vi "modbusTimestampInstruction.vi"(8 "error in (no error)":errorcluster, 11 "Model in":refnum<class "Model.lvclass">) -> (0 "error out":errorcluster, 3 "Model out":refnum<class "Model.lvclass">)   [LabVIEW 2016, in "Model.lvclass"]
uses:
  Model.lvclass
  Model.lvclass/Model.ctl
  ILCCommunications/ILCCommunications.lvclass
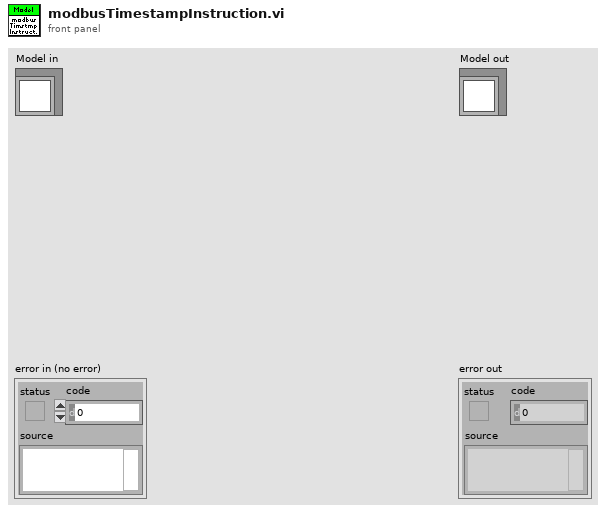
[diagram p1: front panel]
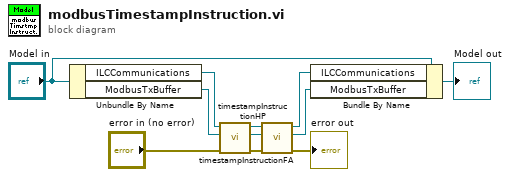
[diagram p0: block diagram]
diagram:
  n1 = Unbundle By Name("Model in") -> ("ILCCommunications"=w9:refnum<class "ILCCommunications.lvclass">, "ModbusTxBuffer"=w8:refnum<class "ModbusBuffer.lvclass">)
  n2 = call "timestampInstructionHP.vi"("error in (no error)"="error in (no error)", "ModbusBuffer in"=w8, "ILCCommunications in"=w9) -> ("error out"=w4:errorcluster, "ModbusBuffer out"=w5:refnum<class "ModbusBuffer.lvclass">, "ILCCommunications out"=w6:refnum<class "ILCCommunications.lvclass">)  [unwired: 6 in]
  n3 = call "timestampInstructionFA.vi"("error in (no error)"=w4, "ModbusBuffer in"=w5, "ILCCommunications in"=w6) -> ("error out"=→"error out":errorcluster, "ModbusBuffer out"=w2:refnum<class "ModbusBuffer.lvclass">, "ILCCommunications out"=w1:refnum<class "ILCCommunications.lvclass">)  [unwired: 6 in]
  n4 = Bundle By Name(cluster="Model in", "ILCCommunications"=w1, "ModbusTxBuffer"=w2) -> (→"Model out":refnum<class "Model.lvclass">)
